vi "IMAGE TO BITSv2.vi"() -> ()   [LabVIEW 2013]
panel:
  out "VHDL":string
  out "Y":i32
  out "X":i32
  out "new picture":picture
  out "Array":string[][](array[string])
  in  "Path":path=path "C:/VIVADO_PROJECTS/VLAK/00GRAPHICS/TEST2.png"
  # "feed PNG picture 24bit color depth without transparency"
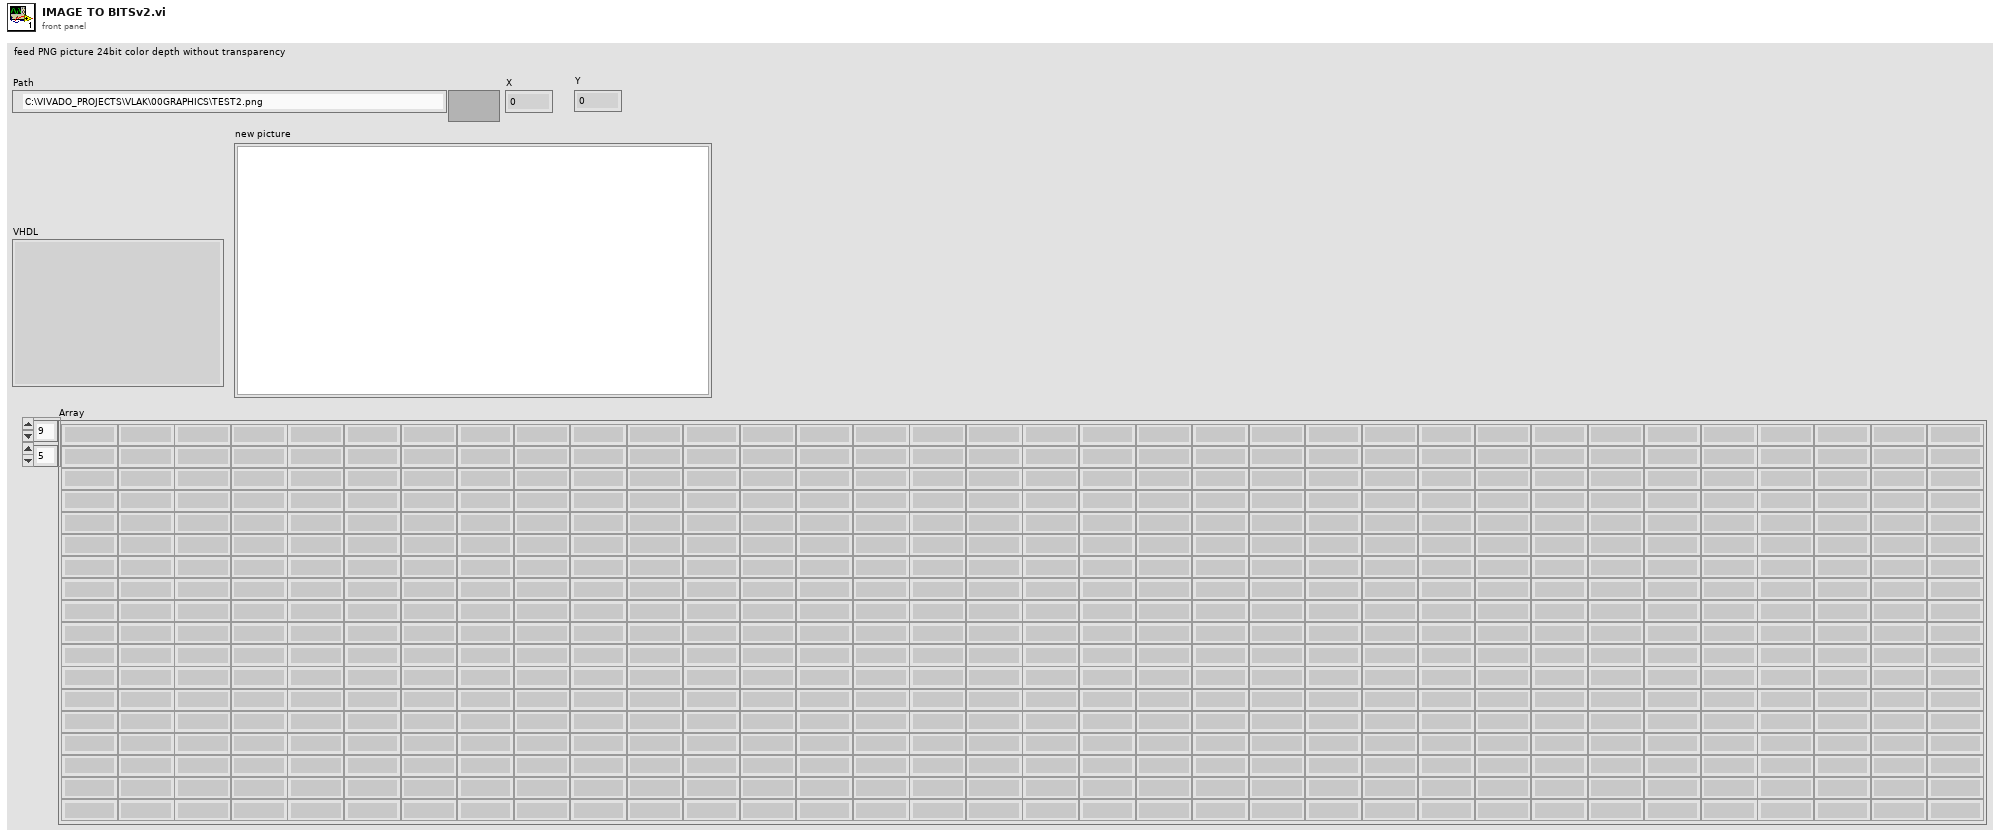
[diagram p1: front panel]
types:
  T1 = typedef "imagedata.ctl" = cluster{"image type":i32, "image depth":i32, "image":u8[], "mask":u8[], "colors":u32[], "Rectangle":cluster{"left":i16, "top":i16, "right":i16, "bottom":i16}}
  T2 = cluster{"left":i16, "top":i16, "right":i16, "bottom":i16}
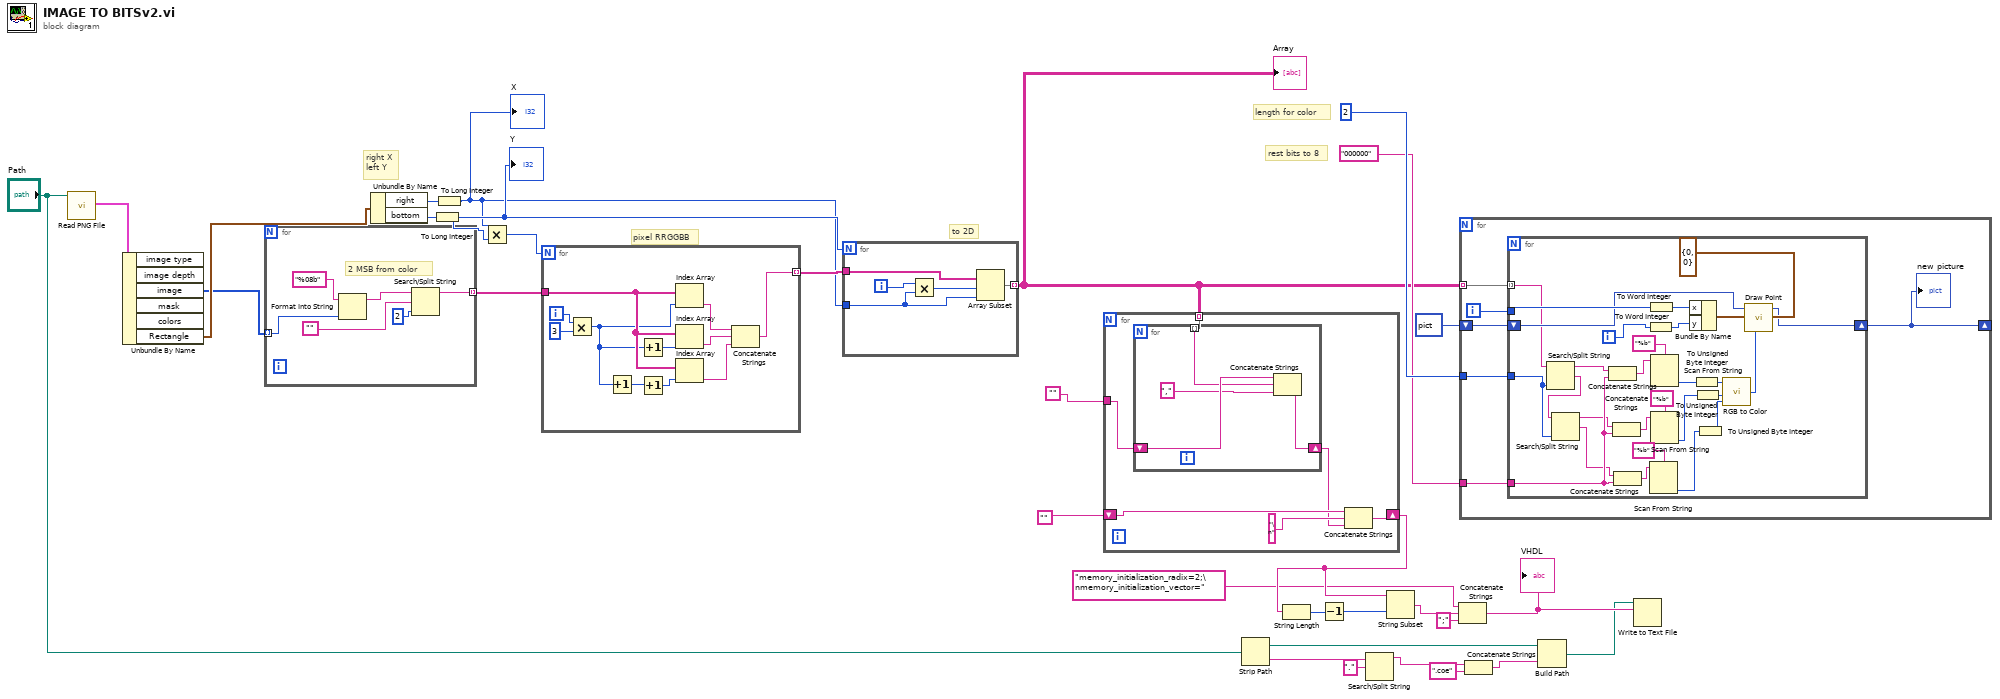
[diagram p0: block diagram]
diagram:
  # "rest bits to 8"
  # "length for color"
  # "right X\nleft Y"
  # "pixel RRGGBB"
  # "to 2D"
  n1 = call <vilib>:"Read PNG File.vi"("path to PNG file"="Path") -> ("image data"=w31:T1)  [unwired: 8 in, 2 out]
  n2 = Unbundle By Name(w31) -> ("image"=w29:u8[], "Rectangle"=w30:T2)  [unwired: 4 out]
  n3 = for {
    tunnel: w29 -> [w36] mode=indexing
    tunnel: [w32] -> w28 mode=indexing
    # "2 MSB from color"
    n4 = Format Into String(format string="%08b", w36) -> (resulting string=w35:string)  [unwired: 2 in, 1 out]
    n5 = Search/Split String(string=w35, search string/char (-)="", offset (0)=2) -> (substring before match=w32:string)  [unwired: 2 out]
  }
  n6 = Unbundle By Name(w30) -> ("right"=w25:i16, "bottom"=w26:i16)
  n7 = To Long Integer(number=w26) -> (32bit integer=w7:i32)
  "Y" <- w7
  n8 = To Long Integer(number=w25) -> (32bit integer=w6:i32)
  "X" <- w6
  n9 = Multiply(x=w6, y=w7) -> (x*y=w10:i32)
  n10 = for {
    N: w10 -> [_]
    tunnel: w28 -> [w48]
    tunnel: [w38] -> w27 mode=indexing
    i -> [w44]
    n11 = Multiply(x=w44, y=3) -> (x*y=w40:i32)
    n12 = Increment(x=w40) -> (x+1=w39:i32)
    n13 = Increment(x=w40) -> (x+1=w42:i32)
    n14 = Increment(x=w39) -> (x+1=w41:i32)
    n15 = Index Array(array=w48, index=w40) -> (element=w47:string)
    n16 = Index Array(array=w48, index=w42) -> (element=w46:string)
    n17 = Index Array(array=w48, index=w41) -> (element=w45:string)
    n18 = Concatenate Strings(w47, w46, w45) -> (w38:string)
  }
  n19 = for {
    N: w7 -> [_]
    tunnel: w6 -> [w53]
    tunnel: w27 -> [w50]
    tunnel: [w49] -> w5 mode=indexing
    i -> [w52]
    n20 = Multiply(x=w52, y=w53) -> (x*y=w51:i32)
    n21 = Array Subset(array=w50, index=w51, length=w53) -> (w49:string[])
  }
  "Array" <- w5
  n22 = for {
    tunnel: w5 -> [w59] mode=indexing
    tunnel: "" -> [w58]
    shift-right: [w54] -> w4
    shift-left: "" -> [w57]
    n23 = for {
      tunnel: w59 -> [w61] mode=indexing
      shift-right: [w62] -> w55
      shift-left: w58 -> [w63]
      n24 = Concatenate Strings(w63, w61, "," ("string")) -> (w62:string)
    }
    n25 = Concatenate Strings(w57, "\n" ("string"), w55) -> (w54:string)
  }
  n26 = Strip Path(path="Path") -> (stripped path=w17:path, name=w16:string)
  n27 = String Length(string=w4) -> (length=w9:i32)
  n28 = Decrement(x=w9) -> (x-1=w8:i32)
  n29 = Search/Split String(string=w16, search string/char (-)=".") -> (substring before match=w14:string)  [unwired: 1 in, 2 out]
  n30 = String Subset(string=w4, length (rest)=w8) -> (substring=w20:string)  [unwired: 1 in]
  n31 = Concatenate Strings("memory_initialization_radix=2;\nmemory_initialization_vector=" ("string"), w20, ";" ("string")) -> (w18:string)
  "VHDL" <- w18
  n32 = for {
    tunnel: w5 -> [w69] mode=indexing
    shift-right: [w67] -> _
    shift-left: picture data[5B] ("new picture") -> [w66]
    tunnel: 2 ("index") -> [w65]
    tunnel: "000000" ("string") -> [w64]
    i -> [w68]
    n33 = for {
      tunnel: w69 -> [w79] mode=indexing
      tunnel: w68 -> [w92]
      shift-right: [w90] -> w67
      shift-left: w66 -> [w89]
      tunnel: w65 -> [w77]
      tunnel: w64 -> [w76]
      i -> [w91]
      n34 = Search/Split String(string=w79, offset (0)=w77) -> (substring before match=w75:string, match + rest of string=w78:string)  [unwired: 1 in, 1 out]
      n35 = Search/Split String(string=w78, offset (0)=w77) -> (substring before match=w73:string, match + rest of string=w71:string)  [unwired: 1 in, 1 out]
      n36 = Concatenate Strings(w75, w76) -> (w74:string)
      n37 = Concatenate Strings(w73, w76) -> (w72:string)
      n38 = Concatenate Strings(w71, w76) -> (w70:string)
      n39 = To Word Integer(number=w91) -> (16bit integer=w94:i16)
      n40 = To Word Integer(number=w92) -> (16bit integer=w93:i16)
      n41 = Scan From String(format string="%b", input string=w70) -> (output 1=w80:i32)  [unwired: 3 in, 3 out]
      n42 = Scan From String(format string="%b", input string=w74) -> (output 1=w84:i32)  [unwired: 3 in, 3 out]
      n43 = Scan From String(format string="%b", input string=w72) -> (output 1=w81:i32)  [unwired: 3 in, 3 out]
      n44 = Bundle By Name(cluster=cluster{"y":i16, "x":i16} {"y"=0, "x"=0} ("point(x,y)"), "x"=w93, "y"=w94) -> (w95:cluster{"y":i16, "x":i16})
      n45 = To Unsigned Byte Integer(number=w84) -> (unsigned 8bit integer=w87:u8)
      n46 = To Unsigned Byte Integer(number=w81) -> (unsigned 8bit integer=w85:u8)
      n47 = To Unsigned Byte Integer(number=w80) -> (unsigned 8bit integer=w86:u8)
      n48 = call <vilib>:"RGB to Color.vi"("B"=w86, "G"=w85, "R"=w87) -> ("Color"=w97:u32)
      n49 = call <vilib>:"Draw Point.vi"("picture"=w89, "point(x,y)"=w95, "color(black)"=w97) -> ("new picture"=w90:picture)  [unwired: 6 in]
    }
    "new picture" <- w67
  }
  n50 = Concatenate Strings(w14, ".coe" ("string")) -> (w12:string)
  n51 = Build Path(base path=w17, name or relative path=w12) -> (appended path=w11:path)
  n52 = Write to Text File(file (use dialog)=w11, text=w18) -> ()  [unwired: 2 in, 3 out]
